vi "Prompt Build Key Array for Config.vi"(8 "error in (no error)":errorcluster, 9 "Prompt Test Parameters":T2, 10 "Key Array In":T3, 11 "Connection Refnum":T1) -> (0 "error out":errorcluster, 1 "$$INITCODE$$":string, 2 "Key Array Out":T3, 3 "Connection Refnum":T1)   [LabVIEW 2011]
uses:
  Addons/internet/utils/keyedarr.llb/Keyed Array.ctl
  TypeDefs/Prompt Test Parameters.ctl
  SI.LIB/ODBC/SQL Controls/Connection Refnum.ctl
  Addons/internet/utils/strutil.llb/Case Matching.ctl
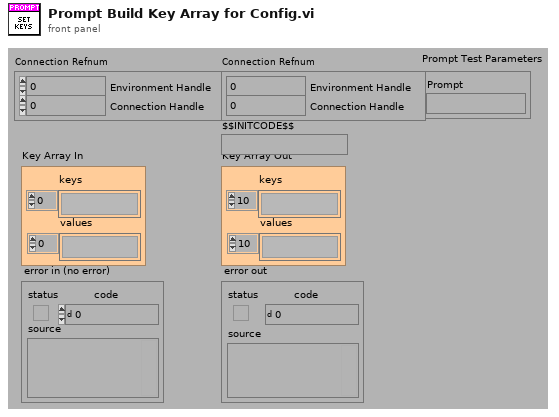
[diagram p1: front panel]
types:
  T1 = typedef "Connection Refnum.ctl" = cluster{"Environment Handle":i32, "Connection Handle":i32}
  T2 = typedef "Prompt Test Parameters.ctl" = cluster{"Prompt":string}
  T3 = typedef "Keyed Array.ctl" = cluster{"keys":string[], "values":string[]}
  T4 = typedef "Case Matching.ctl" = enum16{"a != A", "a == A", "system"}
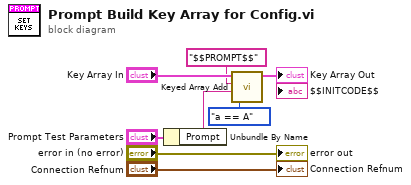
[diagram p0: block diagram]
diagram:
  n1 = Unbundle By Name("Prompt Test Parameters") -> ("Prompt"=w2:string)
  n2 = call "Keyed Array Add.vi"("case matching (sensitive)"=Case_Matching."a == A", "value"=w2, "key"="$$PROMPT$$", "array in"="Key Array In") -> ("array out"=→"Key Array Out":T3)  [unwired: 3 out]
  "error out" <- "error in (no error)"
  "Connection Refnum" <- "Connection Refnum"
